vi "partial_fit.vi"(8 "error in (no error)":errorcluster caption="entrée d'erreur (pas d'erreur)", 11 "PassiveAggressiveRegressor.lvclass 2":refnum<class "PassiveAggressiveRegressor.lvclass">) -> (0 "error out":errorcluster caption="sortie d'erreur", 3 "PassiveAggressiveRegressor.lvclass":refnum<class "PassiveAggressiveRegressor.lvclass">)   [LabVIEW 2020, in "PassiveAggressiveRegressor.lvclass"]
doc: "Fit linear model with Passive Aggressive algorithm.\n\n Parameters\n ----------\n X : {array-like, sparse matrix} of shape (n_samples, n_features)\n Subset of training data\n\n y : numpy array of shape [n_samples]\n Subset of target values\n\n Returns\n -------\n self : returns an instance of self."
uses:
  PassiveAggressiveRegressor.lvclass
  C:/Users/cipop/TDF Dropbox/2_Technologies de France/1 - Services et Etudes/PLAIY/2 - DEV/PLAIYLAB/code/Python/Python.lvclass
  C:/Users/cipop/TDF Dropbox/2_Technologies de France/1 - Services et Etudes/PLAIY/2 - DEV/PLAIYLAB/code/Model/Model.lvclass
  PassiveAggressiveRegressor.lvclass/PassiveAggressiveRegressor.ctl
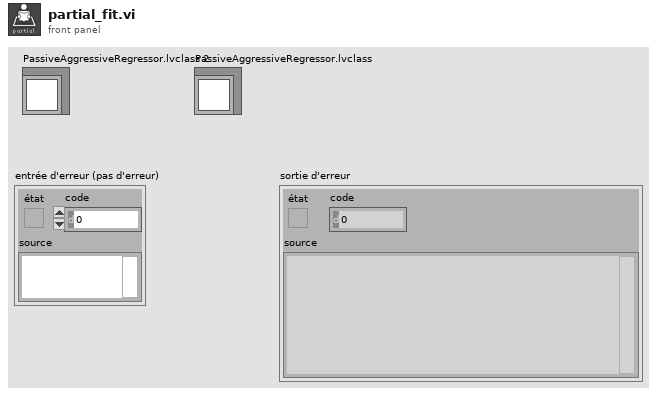
[diagram p1: front panel]
types:
  T1 = typedef "data.ctl" = cluster{"name":string, "X":dbl[][]}
  T2 = typedef "passive_agressive_regressor_data.ctl" = cluster{"y":dbl[], "sample_weight":dbl[], "intercept_init":dbl[], "coef_init":dbl[][]}
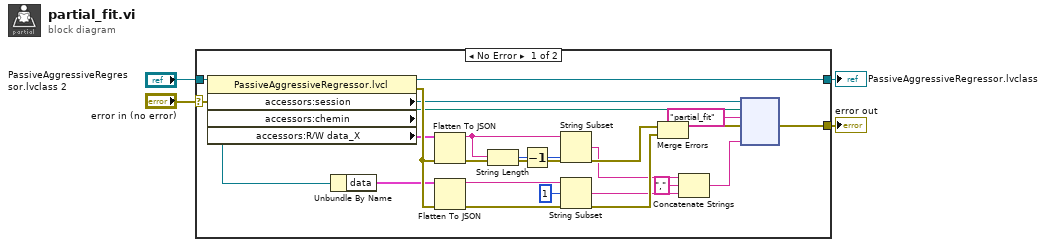
[diagram p0: block diagram]
diagram:
  n1 = case shown="No Error" "error in (no error)" {
    selector: "error in (no error)" -> [w24 w28]
    tunnel: [w25 w28] -> w3
    tunnel: [w7 w27] -> w1
    tunnel: "PassiveAggressiveRegressor.lvclass 2" -> [w6 w27]
    frame No Error {
      n2 = property class="PassiveAggressiveRegressor.lvcl"(reference=w6, error in=w24) -> (reference out=w7:refnum<class "PassiveAggressiveRegressor.lvclass">, error out=w20:errorcluster, "accessors:session"=w10:refnum<k35>, "accessors:chemin"=w9:path, "accessors:R/W data_X"=w11:T1)
      n3 = Unbundle By Name(w6) -> ("data"=w5:T2)
      n4 = Flatten To JSON(anything=w11, error in (no error)=w20) -> (JSON string=w21:string, 11:w16:errorcluster)  [unwired: 1 in]
      n5 = Flatten To JSON(anything=w5, error in (no error)=w20) -> (JSON string=w18:string, 11:w17:errorcluster)  [unwired: 1 in]
      n6 = String Length(string=w21) -> (length=w23:i32)
      n7 = Decrement(x=w23) -> (x-1=w22:i32)
      n8 = String Subset(string=w21, length (rest)=w22) -> (substring=w14:string)  [unwired: 1 in]
      n9 = String Subset(string=w18, offset (0)=1) -> (substring=w13:string)  [unwired: 1 in]
      n10 = Merge Errors(w16, w17) -> (w8:errorcluster)
      n11 = Concatenate Strings(w14, "," ("string"), w13) -> (w12:string)
      n12 = node(w10, w9, "partial_fit" ("nom de la fonction"), w8, w12) -> (w25:errorcluster)  [unwired: 3 in, 3 out]
    }
    frame Error {
    }
  }
  "error out" <- w3
  "PassiveAggressiveRegressor.lvclass" <- w1
